vi "x_axis_stepper_motor.vi"(8 "speed":u32(knob) scale=0.0..20.0, 11 "Direction":bool[](array[boolean])) -> ()   [LabVIEW 2016]
uses:
  <vilib>/DigilentWF/DigilentWF.lvlib
panel:
  # "This program is turn x-axis stepper motor with one step only.\n The x-axis is rotated the egg with horizontal.\nThis stepper motor driven by a A4988 driver with 1/16 resolution.  \nThe  digital I/O pin 0 of Analog Discovery 2 is connected to the enable pin of A4988 driver with implement low logic level.\nThe  digital I/O pin 1 of Analog Discovery 2 is connected to the step pin of A4988 driver with implement a pulse.\nThe  digital I/O pin 2 of Analog Discovery 2 is connected to the direction pin of A4988 driver the value will be input the by user (low logic level or high logic lovel).\nThe  digital I/O pin 3 to 5 of Analog Discovery 2 is connected to the mirco-stepping pin of A4988 driver with implement the all high logic lovel."
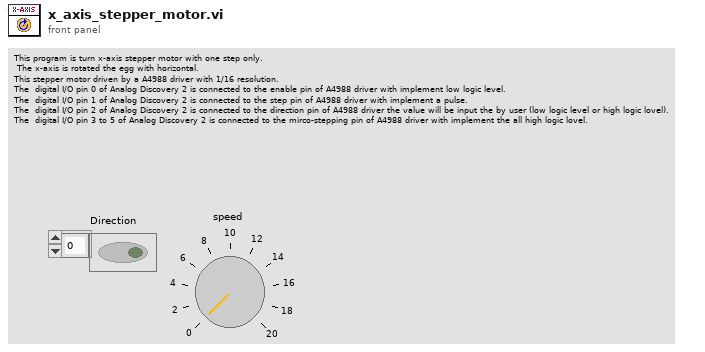
[diagram p1: front panel]
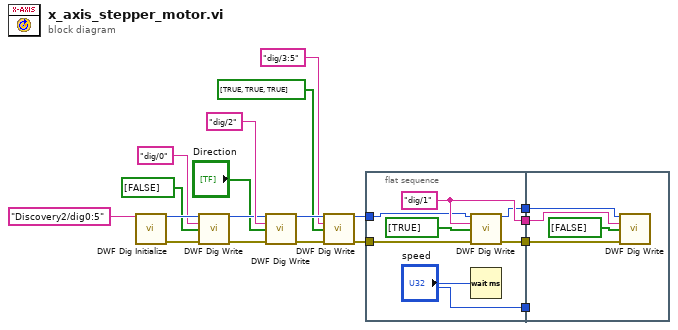
[diagram p0: block diagram]
diagram:
  n1 = call <vilib>:"DWF Dig Initialize.vi"("Device Name/Lines"="Discovery2/dig0:5") -> ("Instrument Handle Out"=w18:u32, "Error Out"=w17:errorcluster)  [unwired: 13 in]
  n2 = call <vilib>:"DWF Dig Write.vi"("Instrument Handle In"=w18, "Lines"="dig/0" ("Disable line"), "Data"=bool[] [FALSE] ("disable"), "Error In"=w17) -> ("Instrument Handle Out"=w10:u32, "Error Out"=w9:errorcluster)  [unwired: 10 in]
  n3 = call <vilib>:"DWF Dig Write.vi"("Instrument Handle In"=w10, "Lines"="dig/2" ("Direction line"), "Data"="Direction", "Error In"=w9) -> ("Instrument Handle Out"=w8:u32, "Error Out"=w7:errorcluster)  [unwired: 10 in]
  n4 = call <vilib>:"DWF Dig Write.vi"("Instrument Handle In"=w8, "Lines"="dig/3:5" ("Microstepping line"), "Data"=bool[] [TRUE, TRUE, TRUE] ("microstepping"), "Error In"=w7) -> ("Instrument Handle Out"=w6:u32, "Error Out"=w5:errorcluster)  [unwired: 10 in]
  n5 = flat-sequence {
    tunnel: [w25] -> w16
    tunnel: w6 -> [w24]
    tunnel: w5 -> [w23]
    tunnel: [w22] -> w15
    tunnel: [w21] -> w14
    tunnel: ["speed"] -> w13
    tunnel: w16 -> [w29]
    tunnel: w15 -> [w28]
    tunnel: w14 -> [w27]
    tunnel: w13 -> [_]
    frame #0 {
      w25 = "dig/1" ("Step line")
      n6 = call <vilib>:"DWF Dig Write.vi"("Instrument Handle In"=w24, "Lines"=w25, "Data"=bool[] [TRUE], "Error In"=w23) -> ("Instrument Handle Out"=w21:u32, "Error Out"=w22:errorcluster)  [unwired: 10 in]
      n7 = Wait (ms)(milliseconds to wait="speed") -> ()  [unwired: 1 out]
    }
    frame #1 {
      n8 = call <vilib>:"DWF Dig Write.vi"("Instrument Handle In"=w27, "Lines"=w29, "Data"=bool[] [FALSE], "Error In"=w28) -> ()  [unwired: 10 in, 2 out]
    }
  }
